vi "CalcSNS.vi"(10 "Load Sensors":dbl[](array[numeric]), 11 "Ref Sensor":dbl) -> (3 "delta SNS":dbl)   [LabVIEW 2013]
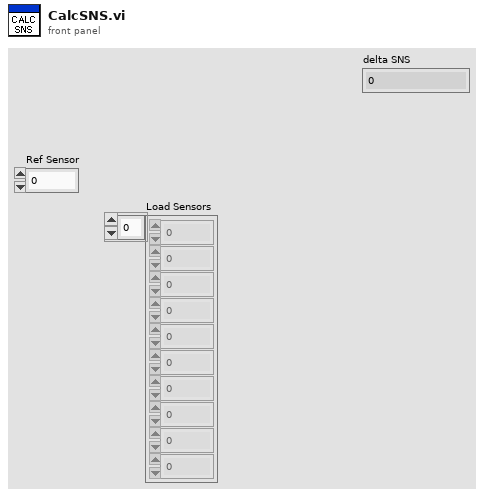
[diagram p1: front panel]
types:
  T1 = cluster{"SNS":dbl, "delta SNS":dbl, "zero SNS":dbl}
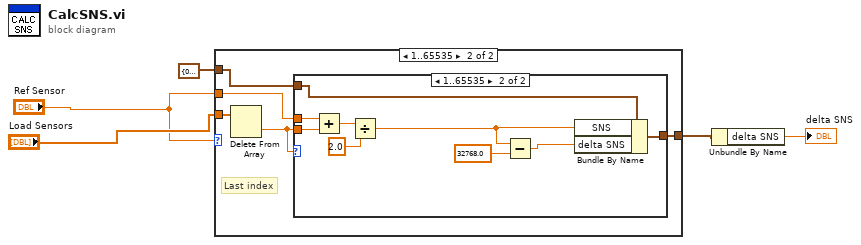
[diagram p0: block diagram]
diagram:
  n1 = case shown="1..65535" "Ref Sensor" {
    tunnel: "Ref Sensor" -> [_ w11]
    tunnel: "Load Sensors" -> [_ w10]
    tunnel: [w6 w9] -> w4
    tunnel: T1 {"SNS"=0.0, "delta SNS"=0.0, "zero SNS"=0.0} ("SNS") -> [w6 w7]
    frame 0, Default {
    }
    frame 1..65535 {
      # "Last index"
      n2 = Delete From Array(array=w10) -> (deleted portion=w8:dbl)  [unwired: 2 in, 1 out]
      n3 = case shown="1..65535" w8 {
        tunnel: w8 -> [_ w20]
        tunnel: w11 -> [_ w18]
        tunnel: [w12 w16] -> w9
        tunnel: w7 -> [w12 w15]
        frame 0, Default {
        }
        frame 1..65535 {
          n4 = Add(x=w18, y=w20) -> (x+y=w21:dbl)
          n5 = Divide(x=w21, y=2.0) -> (x/y=w14:dbl)
          n6 = Subtract(x=w14, y=32768.0) -> (x-y=w17:dbl)
          n7 = Bundle By Name(cluster=w15, "SNS"=w14, "delta SNS"=w17) -> (w16:T1)
        }
      }
    }
  }
  n8 = Unbundle By Name(w4) -> ("delta SNS"=→"delta SNS":dbl)
